vi "Donate.vi"() -> ()   [LabVIEW 2015]
uses:
  Ctrls/btnDonateViaPaypal.ctl
  <vilib>/Platform/browser.llb/Open URL in Default Browser (string).vi
panel:
  in  "btnPaypal":T1
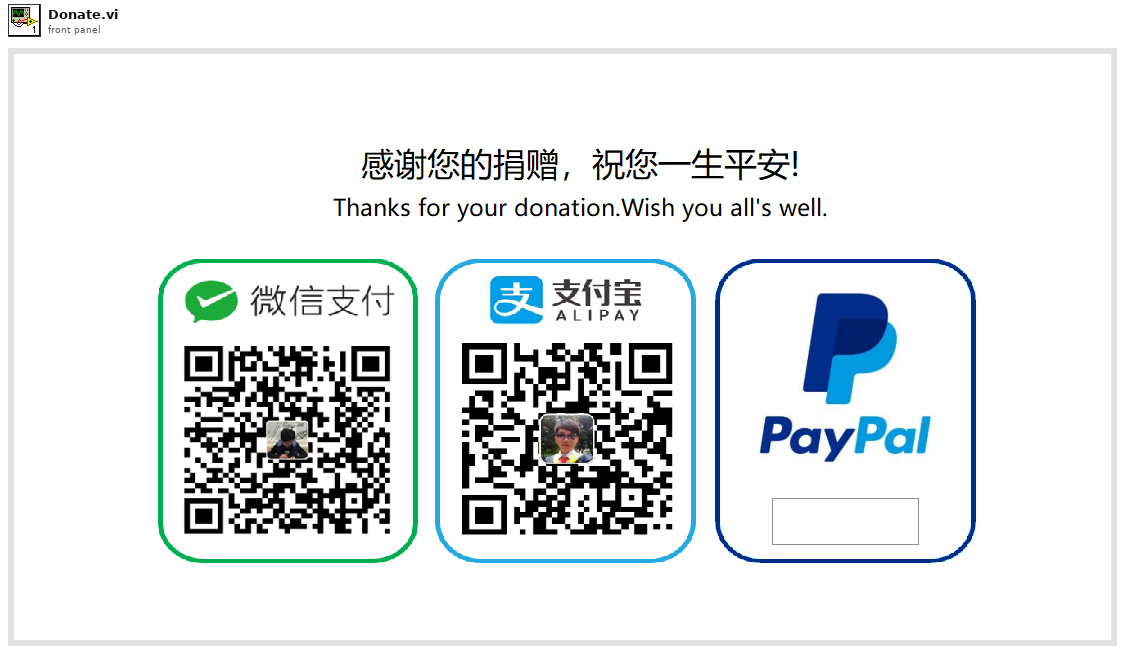
[diagram p1: front panel]
types:
  T1 = typedef "btnDonateViaPaypal.ctl" = bool
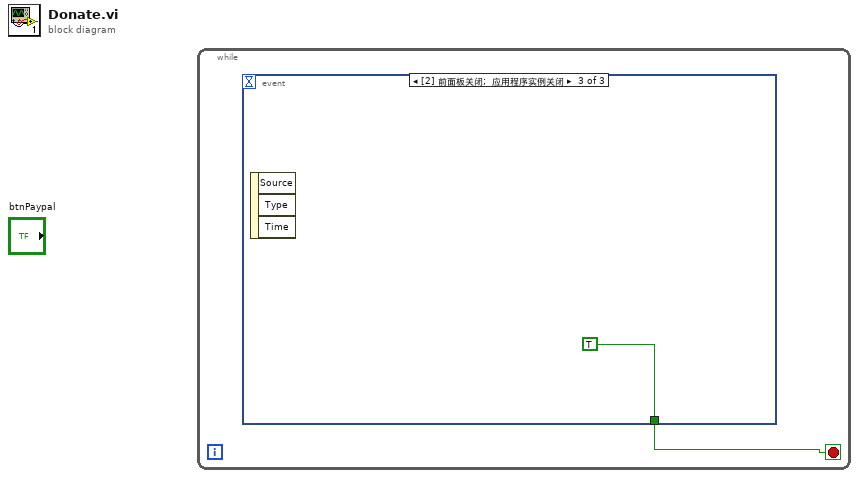
[diagram p0: block diagram]
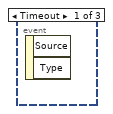
[diagram p2: hidden frame]
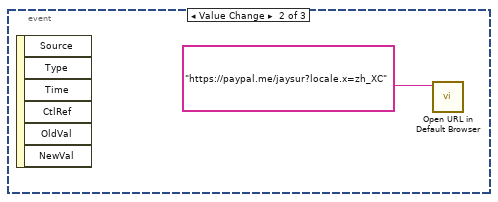
[diagram p3: hidden frame]
diagram:
  n1 = while {
    stop <- w1 stop-if-true
    n2 = event shown="[2] 前面板关闭;  应用程序实例关闭" {
      selector: _ -> [_ _ _]
      dyn-events: _ -> [_ _ _]
      timeout: _ -> [_ _ _]
      tunnel: [_ _ TRUE] -> w1
      event Timeout {
        n3 = event-data() -> ()  [unwired: 1 in, 2 out]
      }
      event Value Change {
        n4 = event-data() -> ()  [unwired: 1 in, 6 out]
        n5 = call-poly <vilib>:"Open URL in Default Browser.vi"("URL"="https://paypal.me/jaysur?locale.x=zh_XC") -> ()  [unwired: 5 in, 2 out]
      }
      event Panel Close; Application Instance Close {
        n6 = event-data() -> ()  [unwired: 1 in, 3 out]
      }
    }
  }
